vi "ADCP_UI_Continuous_Receiver.vi"(8 "error in (no error)":errorcluster, 11 "ADCU_GUI References":T1) -> ()   [LabVIEW 2017]
uses:
  Controls/ADCP_UI/ADCP_UI_Parameters.ctl
  Controls/ADCP_UI/ADCP_UI_Queues.ctl
  Controls/ADCP_UI/ADCP_UI_Continuous_Receiver_States.ctl
  Controls/ADCP_UI/ADCP_Queue_Receive_Log_Queue_Element.ctl
  Controls/Packet/Packet.ctl
  Controls/Packet/Packet_Direction.ctl
  Controls/Packet/Packet_Type.ctl
  Controls/Packet/Packet_Priority.ctl
  Controls/Data Packets/Data_Packet.ctl
  Controls/Data Packets/Parameter.ctl
  Controls/Data Packets/Parameter_Data_Type.ctl
  Controls/Data Packets/Data_Packet_Transmit_Mode.ctl
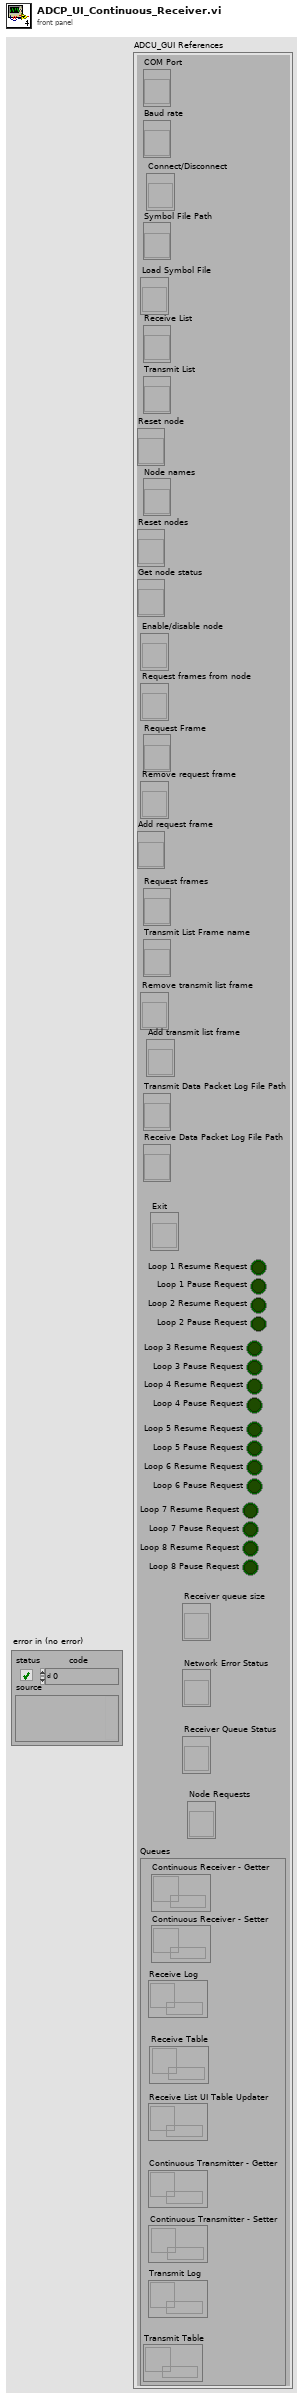
[diagram p1: front panel]
types:
  T1 = typedef "ADCP_UI_Parameters.ctl" = cluster{"COM Port":refnum<vi>, "Baud rate":refnum<vi>, "Symbol File Path":refnum<vi>, "Receive List":refnum<vi>, "Transmit List":refnum<vi>, "Node names":refnum<vi>, "Request Frame":refnum<vi>, "Request frames":refnum<vi>, "Transmit List Frame name":refnum<vi>, "Transmit Data Packet Log File Path":refnum<vi>, "Receive Data Packet Log File Path":refnum<vi>, "Loop 1 Resume Request":bool, "Loop 1 Pause Request":bool, "Loop 2 Resume Request":bool, "Loop 2 Pause Request":bool, "Loop 3 Resume Request":bool, "Loop 3 Pause Request":bool, "Loop 4 Resume Request":bool, "Loop 4 Pause Request":bool, "Loop 5 Resume Request":bool, "Loop 5 Pause Request":bool, "Loop 6 Resume Request":bool, "Loop 6 Pause Request":bool, "Loop 7 Resume Request":bool, "Loop 7 Pause Request":bool, "Loop 8 Resume Request":bool, "Loop 8 Pause Request":bool, "Exit":refnum<vi>, "Connect/Disconnect":refnum<vi>, "Load Symbol File":refnum<vi>, "Reset node":refnum<vi>, "Reset nodes":refnum<vi>, "Get node status":refnum<vi>, "Enable/disable node":refnum<vi>, "Request frames from node":refnum<vi>, "Remove request frame":refnum<vi>, "Add request frame":refnum<vi>, "Remove transmit list frame":refnum<vi>, "Add transmit list frame":refnum<vi>, "Receiver queue size":refnum<vi>, "Network Error Status":refnum<vi>, "Receiver Queue Status":refnum<vi>, "Node Requests":refnum<vi>, "Queues":T2}
  T2 = typedef "ADCP_UI_Queues.ctl" = cluster{"Continuous Receiver - Getter":refnum<queue>, "Continuous Receiver - Setter":refnum<queue>, "Receive Log":refnum<queue>, "Receive Table":refnum<queue>, "Receive List UI Table Updater":refnum<queue>, "Continuous Transmitter - Getter":refnum<queue>, "Continuous Transmitter - Setter":refnum<queue>, "Transmit Log":refnum<queue>, "Transmit Table":refnum<queue>}
  T3 = typedef "ADCP_UI_Continuous_Receiver_States.ctl" = enum16{"Disable", "Enable", "Exit"}
  T4 = typedef "Packet_Direction.ctl" = enum16{"Transmit", "Receive", "Bidirectional"}
  T5 = typedef "ADCP_Queue_Receive_Log_Queue_Element.ctl" = cluster{"Packet":T6, "Receive Time (ms)":u64, "Count":i32, "Receive Time Interval (ms) ":u64}
  T6 = typedef "Packet.ctl" = cluster{"Raw Bytes":u8[], "Checksum":bool, "Direction":T4, "Processed Bytes":u8[], "Node ID":u8, "Packet type":T7, "Frame Data":u32, "Priority":T8, "Frame ID":u8}
  T7 = typedef "Packet_Type.ctl" = enum16{"Data", "Connection Management", "Remote Request", "Error/Status"}
  T8 = typedef "Packet_Priority.ctl" = enum16{"LOW", "HIGH"}
  T9 = typedef "ADCP_UI_Data_Packet_Receiver_Parameters.ctl" = cluster{"Node ID":u32, "Frame ID":u32, "Count":u32, "Last received time (ms)":u32, "Time interval (ms)":u32}
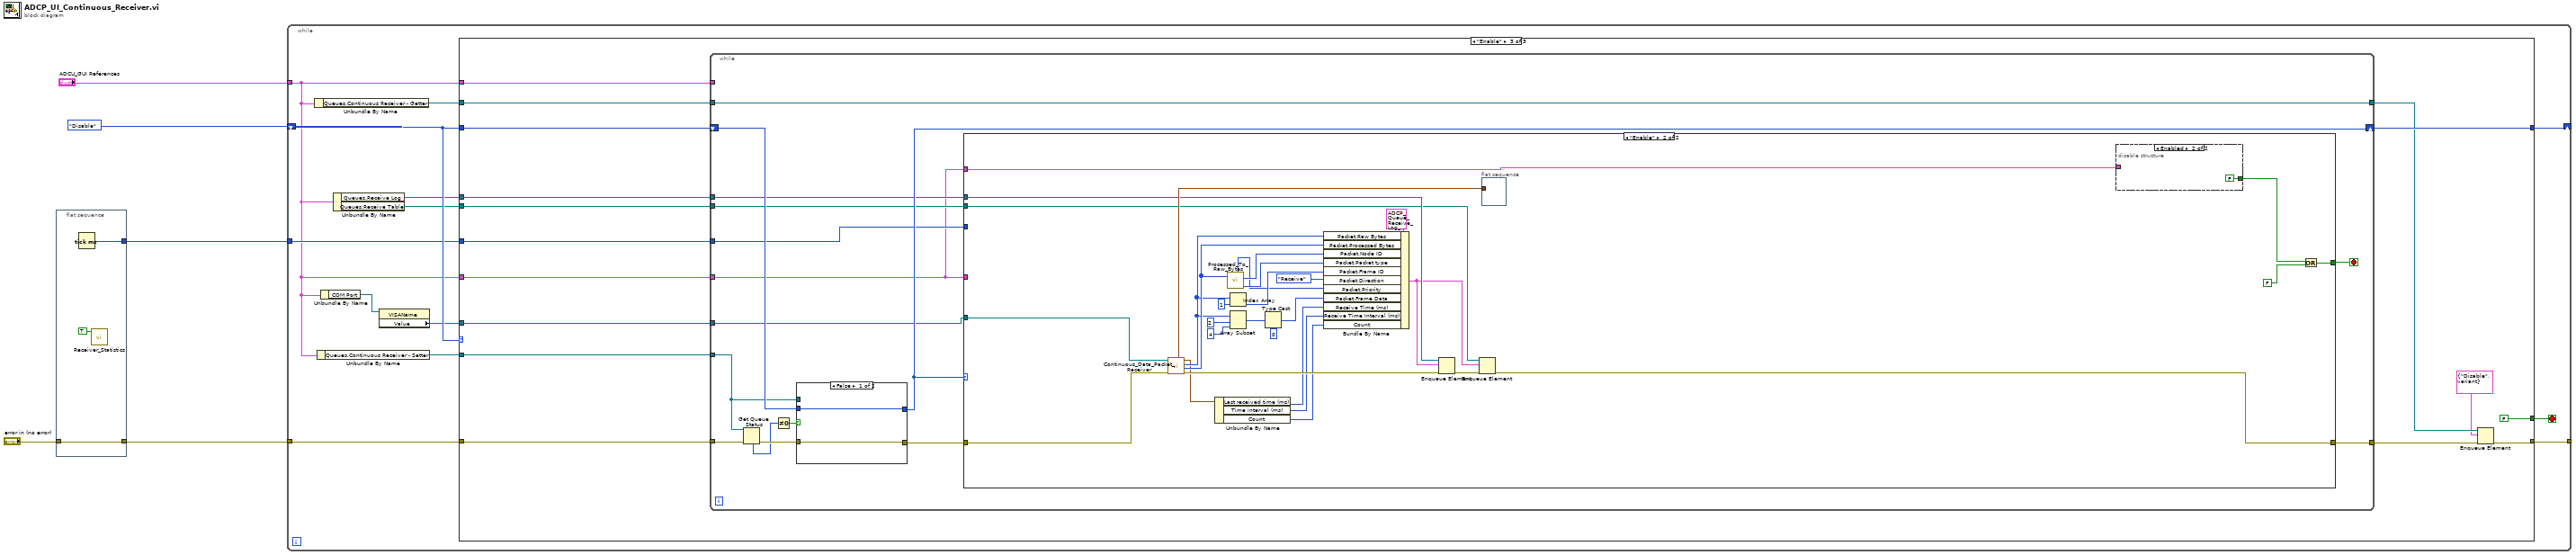
[diagram p0: block diagram]
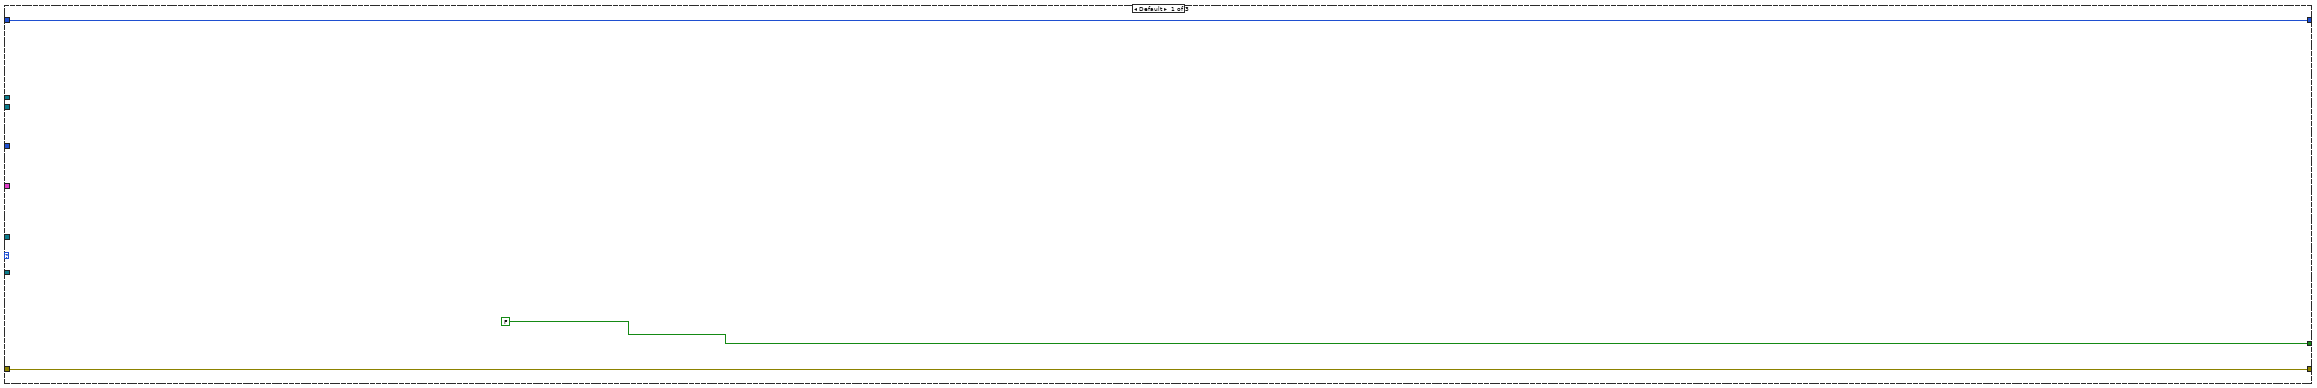
[diagram p2: hidden frame]
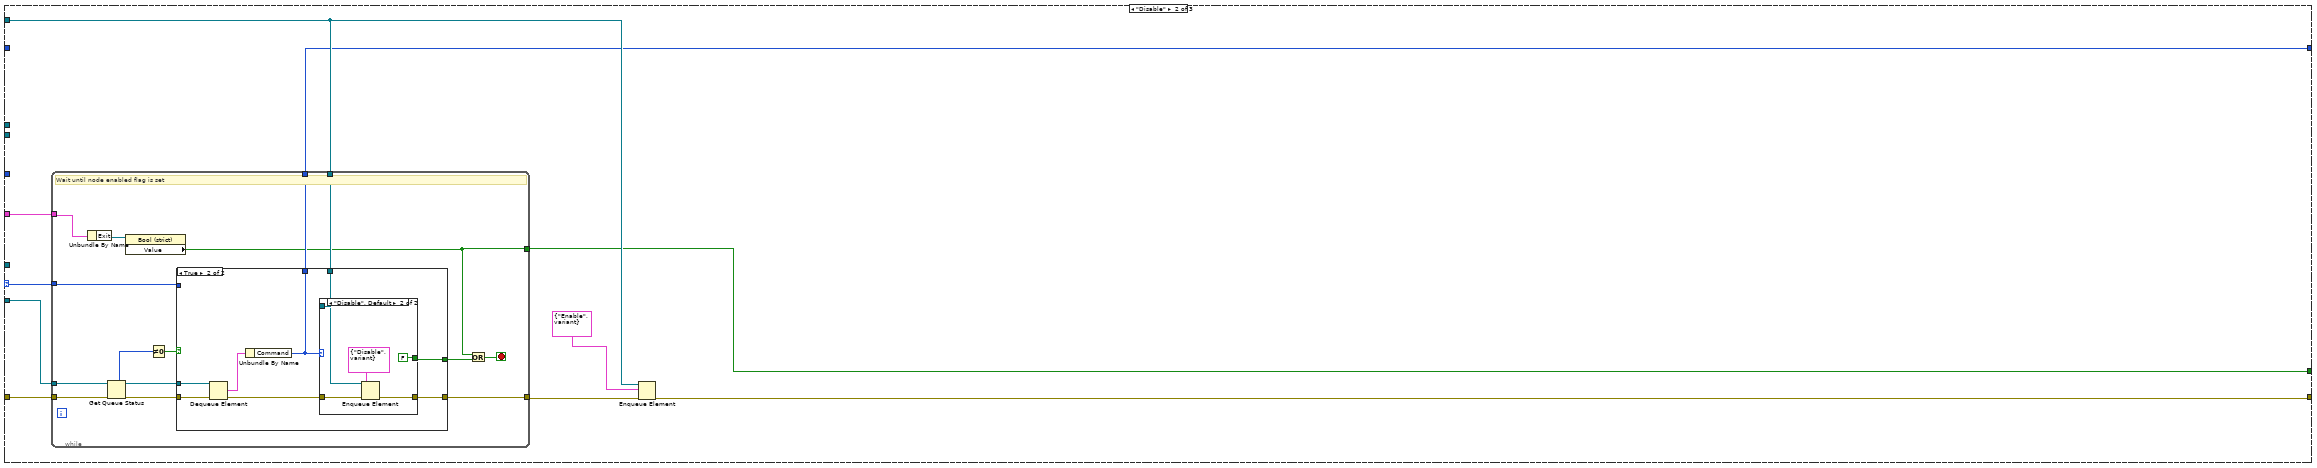
[diagram p3: hidden frame]
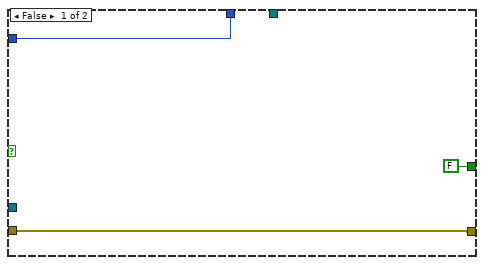
[diagram p4: hidden frame]
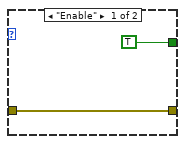
[diagram p5: hidden frame]
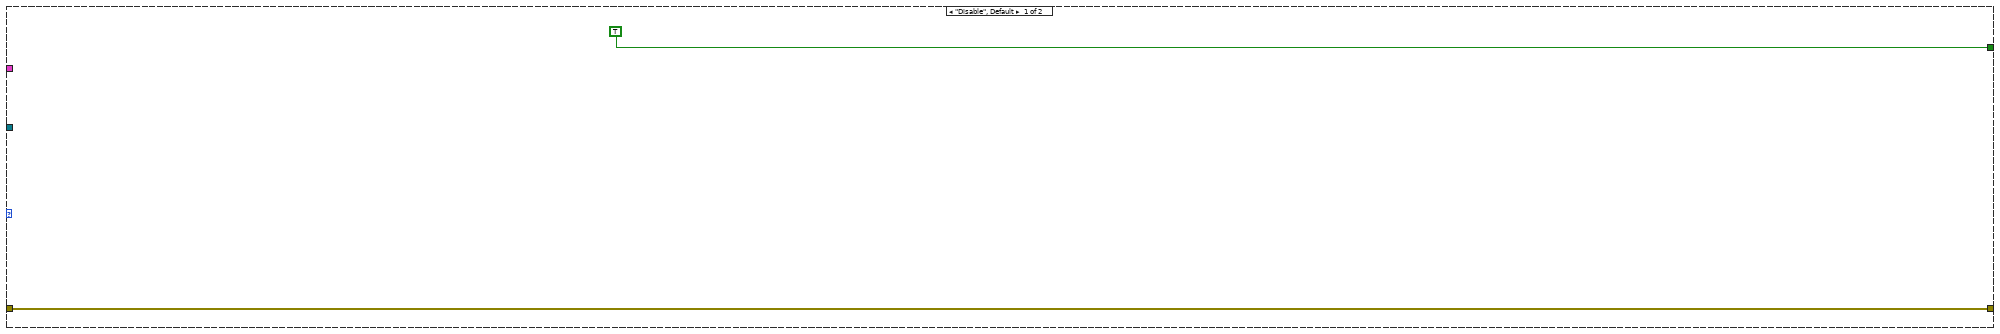
[diagram p6: hidden frame]
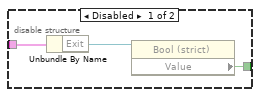
[diagram p7: hidden frame]
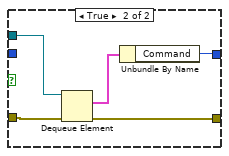
[diagram p8: hidden frame]
diagram:
  n1 = flat-sequence {
    tunnel: "error in (no error)" -> [w8]
    tunnel: [w8] -> w1
    tunnel: [w7] -> w3
    frame #0 {
      n2 = Tick Count (ms)() -> (millisecond timer value=w7:u32)
      n3 = call "Receiver_Statistics.vi"("Initialize ?"=TRUE) -> ()  [unwired: 8 in, 3 out]
    }
  }
  n4 = while {
    tunnel: "ADCU_GUI References" -> [w11]
    tunnel: w1 -> [w19]
    shift-right: [w20] -> _
    shift-left: ADCP_UI_Continuous_Receiver_States."Disable" ("Enum") -> [w21]
    tunnel: [w18] -> _
    tunnel: w3 -> [w14]
    stop <- w17 stop-if-true
    n5 = Unbundle By Name(w11) -> ("Queues.Continuous Receiver - Getter"=w15:refnum<queue>)
    n6 = Unbundle By Name(w11) -> ("Queues.Continuous Receiver - Setter"=w16:refnum<queue>)
    n7 = Unbundle By Name(w11) -> ("COM Port"=w9:refnum<vi>)
    n8 = Unbundle By Name(w11) -> ("Queues.Receive Log"=w13:refnum<queue>, "Queues.Receive Table"=w12:refnum<queue>)
    n9 = property class="VISAName"(reference=w9) -> ("Value"=w10:refnum<visa-resource-name>)  [unwired: 1 in, 2 out]
    n10 = case shown="\"Enable\"" w21 {
      selector: w21 -> [_ w25 _]
      tunnel: w21 -> [w24 _ w80]
      tunnel: [w24 w28 w78] -> w20
      tunnel: w19 -> [w23 w34 w83]
      tunnel: [w23 w31 w75] -> w18
      tunnel: [FALSE w26 FALSE] -> w17
      tunnel: w11 -> [_ _ w82]
      tunnel: w16 -> [_ w33 w81]
      tunnel: w15 -> [_ w29 w77]
      tunnel: w11 -> [_ w27 w69]
      tunnel: w14 -> [_ _ w72]
      tunnel: w13 -> [_ _ w71]
      tunnel: w12 -> [_ _ w70]
      tunnel: w10 -> [_ _ w68]
      frame Default {
      }
      frame "Disable" {
        n11 = while {
          tunnel: w34 -> [w40]
          tunnel: w33 -> [w41]
          tunnel: [w48] -> w32
          tunnel: w29 -> [w49]
          tunnel: [w47] -> w28
          tunnel: w27 -> [w44]
          tunnel: [w42] -> w26
          tunnel: w25 -> [w37]
          stop <- w45 stop-if-true
          # "Wait until node enabled flag is set"
          n12 = Unbundle By Name(w44) -> ("Exit"=w43:refnum<vi>)
          n13 = Get Queue Status(queue=w41, error in (no error)=w40) -> (queue out=w35:refnum<queue>, error out=w39:errorcluster, # elements in queue=w38:i32)  [unwired: 1 in, 5 out]
          n14 = property class="Bool (strict)"(reference=w43) -> ("Value"=w42:bool)  [unwired: 1 in, 2 out]
          n15 = Not Equal To 0?(x=w38) -> (x != 0?=w36:bool)
          n16 = case shown="True" w36 {
            tunnel: w49 -> [_ w58]
            tunnel: [w50 w57] -> w48
            tunnel: [w52 w56] -> w47
            tunnel: [FALSE w55] -> w46
            tunnel: w39 -> [w50 w54]
            tunnel: w37 -> [w52 _]
            tunnel: w35 -> [_ w53]
            frame False {
            }
            frame True {
              n17 = Dequeue Element(queue=w53, error in (no error)=w54) -> (element=w59:cluster{"Command":T3, "Data":variant}, error out=w60:errorcluster)  [unwired: 1 in, 2 out]
              n18 = Unbundle By Name(w59) -> ("Command"=w56:T3)
              n19 = case shown="\"Disable\", Default" w56 {
                tunnel: w60 -> [w62 w67]
                tunnel: w58 -> [_ w66]
                tunnel: [w62 w64] -> w57
                tunnel: [TRUE FALSE] -> w55
                frame "Enable" {
                }
                frame "Disable", Default {
                  n20 = Enqueue Element(queue=w66, element=cluster{"Command":T3, "Data":variant} {"Command"=enum."Disable", "Data"=variant}, error in (no error)=w67) -> (error out=w64:errorcluster)  [unwired: 1 in, 2 out]
                }
              }
            }
          }
          n21 = Or(x=w42, y=w46) -> (x .or. y?=w45:bool)
        }
        n22 = Enqueue Element(queue=w29, element=cluster{"Command":T3, "Data":variant} {"Command"=enum."Enable", "Data"=variant}, error in (no error)=w32) -> (error out=w31:errorcluster)  [unwired: 1 in, 2 out]
      }
      frame "Enable" {
        n23 = while {
          tunnel: w83 -> [w99]
          tunnel: w82 -> [_]
          tunnel: w81 -> [w94]
          shift-right: [w92] -> w78
          shift-left: w80 -> [w95]
          tunnel: [w90] -> w76
          tunnel: w69 -> [w85]
          tunnel: w77 -> [w89]
          tunnel: [w89] -> w74
          tunnel: w72 -> [w88]
          tunnel: w71 -> [w87]
          tunnel: w70 -> [w86]
          tunnel: w68 -> [w84]
          stop <- w91 stop-if-true
          n24 = Get Queue Status(queue=w94, error in (no error)=w99) -> (error out=w98:errorcluster, # elements in queue=w97:i32)  [unwired: 1 in, 6 out]
          n25 = Not Equal To 0?(x=w97) -> (x != 0?=w96:bool)
          n26 = case shown="False" w96 {
            tunnel: w98 -> [w137 w143]
            tunnel: w95 -> [w138 _]
            tunnel: w94 -> [_ w142]
            tunnel: [w137 w140] -> w93
            tunnel: [w138 w139] -> w92
            frame False {
            }
            frame True {
              n27 = Dequeue Element(queue=w142, error in (no error)=w143) -> (element=w141:cluster{"Command":T3, "Data":variant}, error out=w140:errorcluster)  [unwired: 1 in, 2 out]
              n28 = Unbundle By Name(w141) -> ("Command"=w139:T3)
            }
          }
          n29 = case shown="\"Enable\"" w92 {
            tunnel: w93 -> [w100 w127]
            tunnel: [TRUE w131] -> w91
            tunnel: [w100 w104] -> w90
            tunnel: w85 -> [_ _]
            tunnel: w88 -> [_ _]
            tunnel: w87 -> [_ w124]
            tunnel: w86 -> [_ w103]
            tunnel: w85 -> [_ w132]
            tunnel: w84 -> [_ w128]
            frame "Disable", Default {
            }
            frame "Enable" {
              n30 = call "Continuous_Data_Packet_Receiver.vi"("error in (no error)"=w127, "COM Port"=w128) -> ("error out"=w125:errorcluster, "Processed bytes"=w122:u8[], "Raw Bytes"=w117:u8[], "Data Packet Statistics"=w109:T9, "All Data Packet Statistics"=w126:T9[])  [unwired: 5 in]
              n31 = Unbundle By Name(w109) -> ("Last received time (ms)"=w108:u32, "Time interval (ms)"=w107:u32, "Count"=w106:u32)
              n32 = call "Processed_To_Raw_Bytes.vi"("Processed Bytes"=w122) -> ("Packet Type"=w120:T7, "Node ID"=w121:u8, "Priority"=w113:T8)  [unwired: 1 in, 2 out]
              n33 = Index Array(array=w117, index=1) -> (element=w115:u8)
              n34 = Array Subset(array=w117, index=2, length=4) -> (w112:u8[])
              n35 = Type Cast(type=u32 0, x=w112) -> (*(type *) &x=w110:u32)
              n36 = Bundle By Name(cluster=T5 {"Packet"={"Raw Bytes"=[], "Checksum"=FALSE, "Direction"=enum."Transmit", "Processed Bytes"=[], "Node ID"=0, "Packet type"=enum."Data", "Frame Data"=0, "Priority"=enum."LOW", "Frame ID"=0}, "Receive Time (ms)"=0, "Count"=0, "Receive Time Interval (ms) "=0} ("element"), "Packet.Raw Bytes"=w117, "Packet.Processed Bytes"=w122, "Packet.Node ID"=w121, "Packet.Packet type"=w120, "Packet.Frame ID"=w115, "Packet.Direction"=Packet_Direction."Receive", "Packet.Priority"=w113, "Packet.Frame Data"=w110, "Receive Time (ms)"=w108, "Receive Time Interval (ms)"=w107, "Count"=w106) -> (w102:T5)
              n37 = Enqueue Element(queue=w124, element=w102, error in (no error)=w125) -> (error out=w105:errorcluster)  [unwired: 1 in, 2 out]
              n38 = Enqueue Element(queue=w103, element=w102, error in (no error)=w105) -> (error out=w104:errorcluster)  [unwired: 1 in, 2 out]
              n39 = flat-sequence {
                tunnel: w126 -> [_]
                frame #0 {
                }
              }
              n40 = disable-structure shown="Enabled" {
                disable-tunnel: w132 -> [w135 _]
                disable-tunnel: [w133 FALSE ("Value")] -> w130
                frame Disabled {
                  n41 = Unbundle By Name(w135) -> ("Exit"=w134:refnum<vi>)
                  n42 = property class="Bool (strict)"(reference=w134) -> ("Value"=w133:bool)  [unwired: 1 in, 2 out]
                }
                frame Enabled {
                }
              }
              n43 = Or(x=w130, y=FALSE) -> (x .or. y?=w131:bool)
            }
          }
        }
        n44 = Enqueue Element(queue=w74, element=cluster{"Command":T3, "Data":variant} {"Command"=enum."Disable", "Data"=variant}, error in (no error)=w76) -> (error out=w75:errorcluster)  [unwired: 1 in, 2 out]
      }
    }
  }
